vi "ChangeWhileMeasuring.vi"(8 "error in (no error)":errorcluster, 11 "NHRDCPower in":refnum<class "NHRDCPower.lvclass">) -> (0 "error out":errorcluster, 1 "InsturmentSettings":bool, 2 "OutputOrLoadState":bool, 3 "NHRDCPower out":refnum<class "NHRDCPower.lvclass">)   [LabVIEW 2018, in "AcPwrPlugins.lvlib" / "NHRDCPower.lvclass"]
uses:
  NHRDCPower.lvclass
  AcPwrBaseClass/AcPwrBase.lvclass
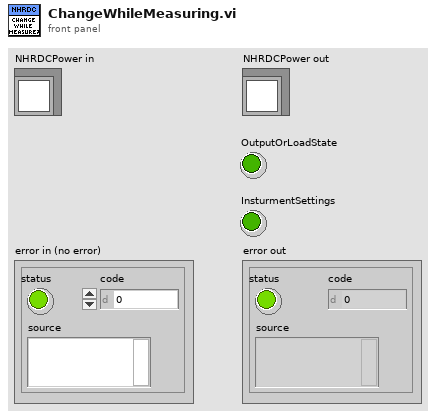
[diagram p1: front panel]
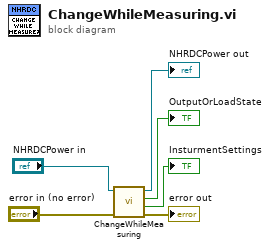
[diagram p0: block diagram]
diagram:
  n1 = call-parent "ChangeWhileMeasuring.vi"("error in (no error)"="error in (no error)", "AcPwrBase in"="NHRDCPower in") -> ("error out"=→"error out":errorcluster, "InsturmentSettings"=→"InsturmentSettings":bool, "OutputOrLoadState"=→"OutputOrLoadState":bool, "AcPwrBase out"=→"NHRDCPower out":refnum<class "NHRDCPower.lvclass">)  [unwired: 6 in]
